vi "MAVLink Command ACK.vi"(7 "FGV Method":T2, 11 "COMMAND ACK":T1) -> (3 "COMMAND ACK out":T1)   [LabVIEW 2014]
uses:
  Controls/FGV Methods.ctl
  MAVLink/Controls/MAVLink Command ACK.ctl
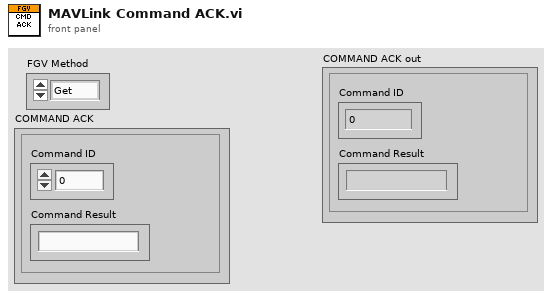
[diagram p1: front panel]
types:
  T1 = typedef "MAVLink Command ACK.ctl" = cluster{"Command ID":u16, "Command Result":string}
  T2 = typedef "FGV Methods.ctl" = enum16{"Get", "Set"}
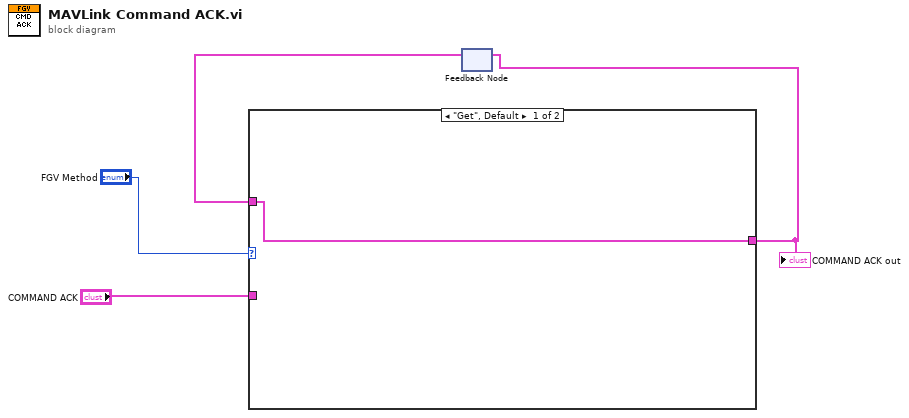
[diagram p0: block diagram]
diagram:
  n1 = feedback #1() -> (w2:T1)  [unwired: 1 in]
  n2 = case shown="\"Get\", Default" "FGV Method" {
    tunnel: "COMMAND ACK" -> [_ w6]
    tunnel: [w5 w6] -> w3
    tunnel: w2 -> [w5 _]
    frame "Get", Default {
    }
    frame "Set" {
    }
  }
  "COMMAND ACK out" <- w3
  n3 = feedback-in #1(w3) -> ()
